vi "Query Vi.vi"(7 "Enum":enum16{"Fetch", "Insert or Update"}(ring)=enum."Insert or Update", 8 "error in (no error)":errorcluster, 10 "SQL query":string, 11 "Refnum in":T2) -> (0 "error out":errorcluster, 3 "recordset reference out":T1, 4 "element":string, 6 "data":string[][](array[string]))   [LabVIEW 2020]
uses:
  <vilib>/addons/database/Connection.llb/Conn ObjectReference.ctl
  <vilib>/addons/database/Recordset.llb/Rec ObjectReference.ctl
  <vilib>/addons/database/Connection.llb/Conn Execute.vi
  <vilib>/addons/database/Recordset.llb/Rec Fetch Recordset Data (R).vi
  <vilib>/addons/database/Recordset.llb/Rec Destroy - Connection.vi
  <vilib>/addons/database/_DB Variant To Data/Database Variant To Data.xnode
  <vilib>/addons/database/NI_Database_API.lvlib
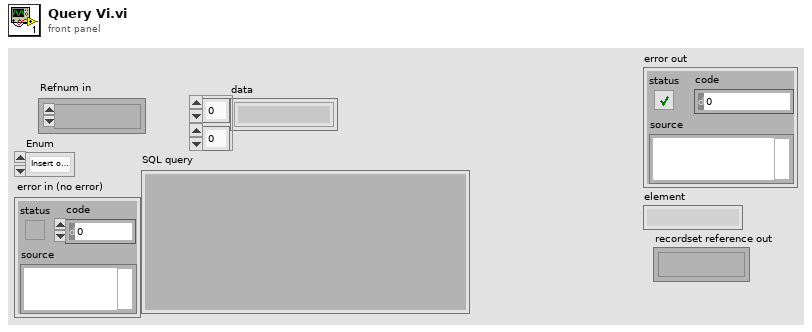
[diagram p1: front panel]
types:
  T1 = typedef "NI_Database_API.lvlib/Rec ObjectReference.ctl" = refnum<k1>
  T2 = typedef "NI_Database_API.lvlib/Conn ObjectReference.ctl" = refnum<k1>
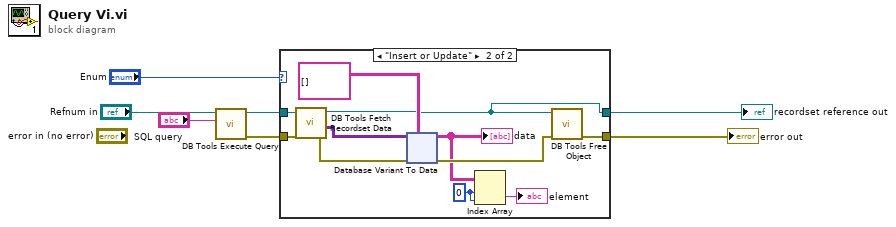
[diagram p0: block diagram]
diagram:
  n1 = call-poly <vilib>:"DB Tools Execute Query.vi"("SQL query"="SQL query", "connection reference"="Refnum in") -> ("error out"=w5:errorcluster, "recordset reference"=w4:T1)  [unwired: 6 in]
  n2 = case shown="\"Insert or Update\"" "Enum" {
    tunnel: w4 -> [w9 w20]
    tunnel: w5 -> [w8 w19]
    tunnel: [w9 w13] -> w2
    tunnel: [w8 w14] -> w3
    frame "Fetch", Default {
    }
    frame "Insert or Update" {
      w11 = 0 ("index (row)")
      n3 = call-poly <vilib>:"DB Tools Fetch Recordset Data.vi"("error in (no error)"=w19, "recordset reference"=w20) -> ("error out"=w17:errorcluster, "recordset data"=w18:variant[][], "recordset reference out"=w13:T1)  [unwired: 3 in]
      n4 = xnode "Database Variant To Data"("database variant"=w18, "error in (no error)"=w17, "type"=string[][] []) -> ("data"=w12:string[][], "error out"=w16:errorcluster)
      "data" <- w12
      n5 = Index Array(array=w12, index (row)=w11, index (col)=w11) -> (element=→"element":string)
      n6 = call-poly <vilib>:"DB Tools Free Object.vi"("error in (no error)"=w16, "recordset reference"=w13) -> ("error out"=w14:errorcluster)  [unwired: 8 in, 1 out]
    }
  }
  "error out" <- w3
  "recordset reference out" <- w2
